vi "bin_to_text.vi"(11 "Boolean in":bool) -> (3 "String":string)   [LabVIEW 2017]
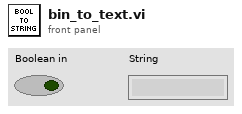
[diagram p1: front panel]
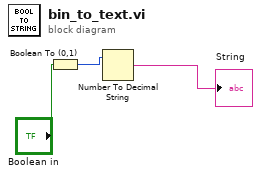
[diagram p0: block diagram]
diagram:
  n1 = Boolean To (0,1)(Boolean="Boolean in") -> (0, 1=w2:i16)
  n2 = Number To Decimal String(number=w2) -> (decimal integer string=→"String":string)  [unwired: 1 in]
